vi "HTS_CUSTOM_WELLS.vi"() -> (2 "Custom Wells":T1[](array[typedef])=[{"Column"=enum."1", "Row"=enum."A"}, {"Column"=enum."2", "Row"=enum."A"}, {"Column"=enum."3", "Row"=enum."A"}, {"Column"=enum."4", "Row"=enum."A"}, {"Column"=enum."5", "Row"=enum."A"}, {"Column"=enum."6", "Row"=enum."A"}, {"Column"=enum."7", "Row"=enum."A"}, {"Column"=enum."1", "Row"=enum."B"}, {"Column"=enum."2", "Row"=enum."B"}, {"Column"=enum."3", "Row"=enum."B"}, {"Column"=enum."4", "Row"=enum."B"}, {"Column"=enum."5", "Row"=enum."B"}, {"Column"=enum."6", "Row"=enum."B"}, {"Column"=enum."7", "Row"=enum."B"}, {"Column"=enum."1", "Row"=enum."C"}, {"Column"=enum."2", "Row"=enum."C"}, {"Column"=enum."3", "Row"=enum."C"}, {"Column"=enum."4", "Row"=enum."C"}, {"Column"=enum."5", "Row"=enum."C"}, {"Column"=enum."6", "Row"=enum."C"}, {"Column"=enum."7", "Row"=enum."C"}, {"Column"=enum."1", "Row"=enum."D"}, {"Column"=enum."2", "Row"=enum."D"}, {"Column"=enum."3", "Row"=enum."D"}, {"Column"=enum."4", "Row"=enum."D"}, {"Column"=enum."5", "Row"=enum."D"}, {"Column"=enum."6", "Row"=enum."D"}, {"Column"=enum."7", "Row"=enum."D"}, {"Column"=enum."1", "Row"=enum."E"}, {"Column"=enum."2", "Row"=enum."E"}, {"Column"=enum."3", "Row"=enum."E"}, {"Column"=enum."4", "Row"=enum."E"}, {"Column"=enum."5", "Row"=enum."E"}, {"Column"=enum."6", "Row"=enum."E"}, {"Column"=enum."7", "Row"=enum."E"}, {"Column"=enum."1", "Row"=enum."F"}, {"Column"=enum."2", "Row"=enum."F"}, {"Column"=enum."3", "Row"=enum."F"}, {"Column"=enum."4", "Row"=enum."F"}, {"Column"=enum."5", "Row"=enum."F"}, {"Column"=enum."6", "Row"=enum."F"}, {"Column"=enum."7", "Row"=enum."F"}, {"Column"=enum."1", "Row"=enum."G"}, {"Column"=enum."2", "Row"=enum."G"}, {"Column"=enum."3", "Row"=enum."G"}, {"Column"=enum."4", "Row"=enum."G"}, {"Column"=enum."5", "Row"=enum."G"}, {"Column"=enum."6", "Row"=enum."G"}, {"Column"=enum."7", "Row"=enum."G"}, {"Column"=enum."1", "Row"=enum."H"}, {"Column"=enum."2", "Row"=enum."H"}, {"Column"=enum."3", "Row"=enum."H"}, {"Column"=enum."4", "Row"=enum."H"}, {"Column"=enum."5", "Row"=enum."H"}, {"Column"=enum."6", "Row"=enum."H"}, {"Column"=enum."7", "Row"=enum."H"}, {"Column"=enum."1", "Row"=enum."A"}])   [LabVIEW 2009]
uses:
  HTS_WELL.ctl
  HTS_COLUMN.ctl
  HTS_ROW.ctl
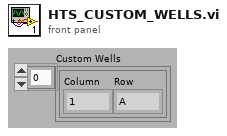
[diagram p1: front panel]
types:
  T1 = typedef "HTS_WELL.ctl" = cluster{"Column":T2, "Row":T3}
  T2 = typedef "HTS_COLUMN.ctl" = enum16{"1", "2", "3", "4", "5", "6", "7", "8", "9", "10", "11", "12"}
  T3 = typedef "HTS_ROW.ctl" = enum16{"A", "B", "C", "D", "E", "F", "G", "H"}
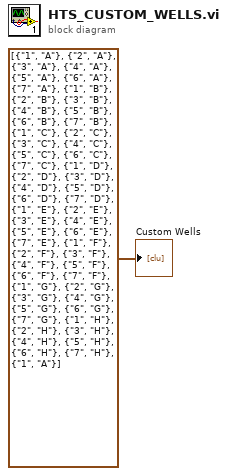
[diagram p0: block diagram]
diagram:
  "Custom Wells" <- T1[] [{"Column"=enum."1", "Row"=enum."A"}, {"Column"=enum."2", "Row"=enum."A"}, {"Column"=enum."3", "Row"=enum."A"}, {"Column"=enum."4", "Row"=enum."A"}, {"Column"=enum."5", "Row"=enum."A"}, {"Column"=enum."6", "Row"=enum."A"}, {"Column"=enum."7", "Row"=enum."A"}, {"Column"=enum."1", "Row"=enum."B"}, {"Column"=enum."2", "Row"=enum."B"}, {"Column"=enum."3", "Row"=enum."B"}, {"Column"=enum."4", "Row"=enum."B"}, {"Column"=enum."5", "Row"=enum."B"}, {"Column"=enum."6", "Row"=enum."B"}, {"Column"=enum."7", "Row"=enum."B"}, {"Column"=enum."1", "Row"=enum."C"}, {"Column"=enum."2", "Row"=enum."C"}, {"Column"=enum."3", "Row"=enum."C"}, {"Column"=enum."4", "Row"=enum."C"}, {"Column"=enum."5", "Row"=enum."C"}, {"Column"=enum."6", "Row"=enum."C"}, {"Column"=enum."7", "Row"=enum."C"}, {"Column"=enum."1", "Row"=enum."D"}, {"Column"=enum."2", "Row"=enum."D"}, {"Column"=enum."3", "Row"=enum."D"}, {"Column"=enum."4", "Row"=enum."D"}, {"Column"=enum."5", "Row"=enum."D"}, {"Column"=enum."6", "Row"=enum."D"}, {"Column"=enum."7", "Row"=enum."D"}, {"Column"=enum."1", "Row"=enum."E"}, {"Column"=enum."2", "Row"=enum."E"}, {"Column"=enum."3", "Row"=enum."E"}, {"Column"=enum."4", "Row"=enum."E"}, {"Column"=enum."5", "Row"=enum."E"}, {"Column"=enum."6", "Row"=enum."E"}, {"Column"=enum."7", "Row"=enum."E"}, {"Column"=enum."1", "Row"=enum."F"}, {"Column"=enum."2", "Row"=enum."F"}, {"Column"=enum."3", "Row"=enum."F"}, {"Column"=enum."4", "Row"=enum."F"}, {"Column"=enum."5", "Row"=enum."F"}, {"Column"=enum."6", "Row"=enum."F"}, {"Column"=enum."7", "Row"=enum."F"}, {"Column"=enum."1", "Row"=enum."G"}, {"Column"=enum."2", "Row"=enum."G"}, {"Column"=enum."3", "Row"=enum."G"}, {"Column"=enum."4", "Row"=enum."G"}, {"Column"=enum."5", "Row"=enum."G"}, {"Column"=enum."6", "Row"=enum."G"}, {"Column"=enum."7", "Row"=enum."G"}, {"Column"=enum."1", "Row"=enum."H"}, {"Column"=enum."2", "Row"=enum."H"}, {"Column"=enum."3", "Row"=enum."H"}, {"Column"=enum."4", "Row"=enum."H"}, {"Column"=enum."5", "Row"=enum."H"}, {"Column"=enum."6", "Row"=enum."H"}, {"Column"=enum."7", "Row"=enum."H"}, {"Column"=enum."1", "Row"=enum."A"}] ("Well Array")
